vi "PathPlanner_Path_BezierFromPoses.vi"(11 "Poses":T2[](array[typedef]) {"ROTATION"."SIN" format="%13.4f"; "ROTATION"."COS" format="%13.4f"; "ROTATION"."VALUE" format="%13.4f"; "TRANSLATION"."Y" format="%14.3f"; "TRANSLATION"."X" format="%14.3f"}) -> (0 "Error":bool, 3 "Bezier":T1[](array[typedef]) {"Y" format="%14.3f"; "X" format="%14.3f"})   [LabVIEW 2019, in "PathPlanner24.lvlib"]
doc: "Create the bezier points necessary to create a path using a list of poses\n\nInputs: \n - poses - pose2d array - List of poses. Each pose represents one waypoint.\n\nOutputs:\n - Bezier - translation2d array - List of bezier points\n - Error - boolean - TRUE if an error occured. (Too few poses)"
uses:
  PathPlanner24.lvlib
  <vilib>/Rock Robotics/WPI/ThirdParty/JAS_Junk/TrajLib/TypeDef/POSE2D.ctl
  <vilib>/Rock Robotics/WPI/ThirdParty/JAS_Junk/TrajLib/TypeDef/TRANSLATION2D.ctl
  <vilib>/Rock Robotics/WPI/ThirdParty/JAS_Junk/TrajLib/TypeDef/ROTATION2D.ctl
  <vilib>/Rock Robotics/WPI/ThirdParty/JAS_Junk/TrajLib/Util_CalcDist.vi
  <vilib>/Rock Robotics/WPI/ThirdParty/JAS_Junk/TrajLib/Rotation2d_GetAngleCosSin.vi
  <vilib>/Rock Robotics/WPI/ThirdParty/JAS_Junk/TrajLib/Translation2d_Create.vi
  <vilib>/Rock Robotics/WPI/ThirdParty/JAS_Junk/TrajLib/Rotation2d_RotateBy.vi
  <vilib>/Rock Robotics/WPI/ThirdParty/JAS_Junk/TrajLib/Conv_Deg_Radians.vi
  <vilib>/Rock Robotics/WPI/ThirdParty/JAS_Junk/TrajLib/Rotation2d_CreateAngle.vi
  <vilib>/Rock Robotics/WPI/ThirdParty/JAS_Junk/TrajLib/Rotation2d_CreateXY.vi
  <vilib>/Rock Robotics/WPI/ThirdParty/JAS_Junk/TrajLib/Trajectory_Library.lvlib
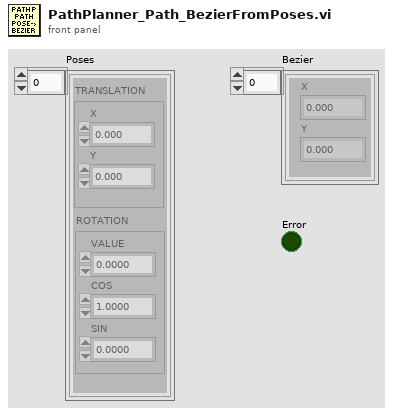
[diagram p1: front panel]
types:
  T1 = typedef "Trajectory_Library.lvlib/TRANSLATION2D.ctl" = cluster{"X":dbl, "Y":dbl}
  T2 = typedef "Trajectory_Library.lvlib/POSE2D.ctl" = cluster{"TRANSLATION":T1, "ROTATION":T3}
  T3 = typedef "Trajectory_Library.lvlib/ROTATION2D.ctl" = cluster{"VALUE":dbl, "COS":dbl, "SIN":dbl}
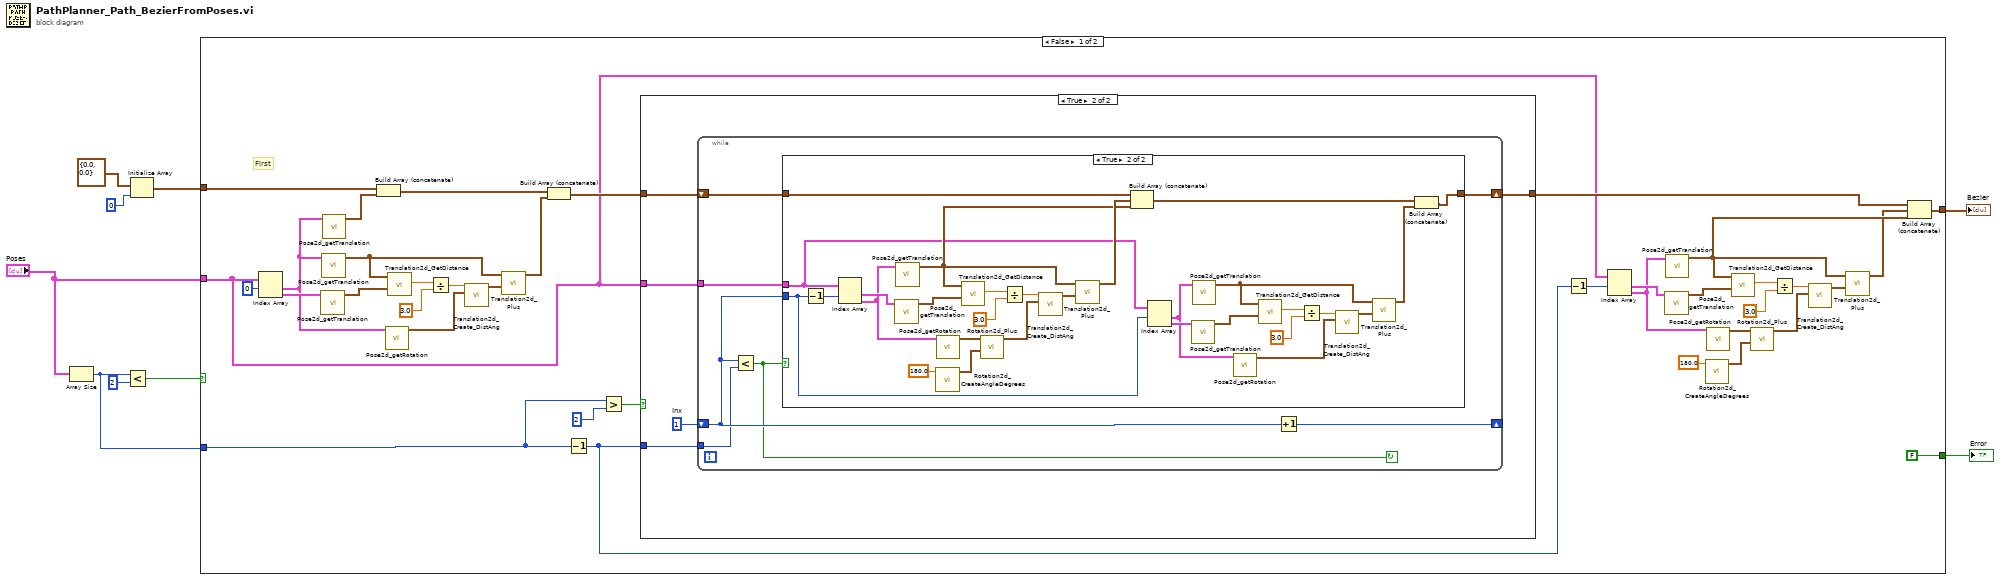
[diagram p0: block diagram]
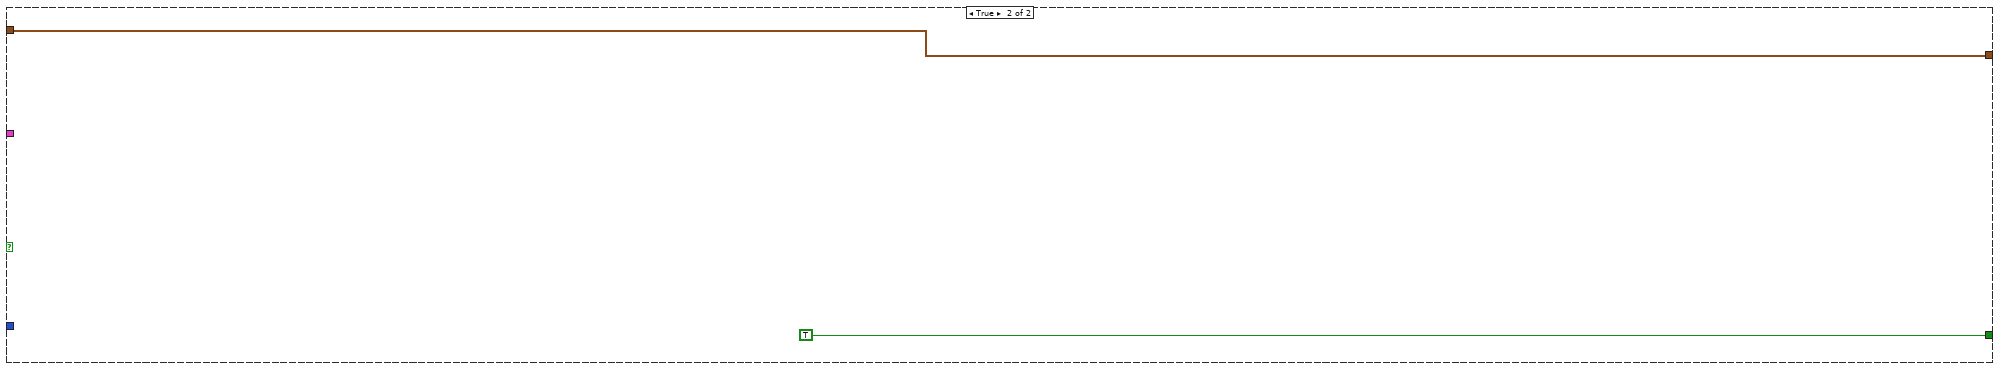
[diagram p4: hidden frame]
diagram:
  n1 = Array Size(array="Poses") -> (size(s)=w2:i32)
  n2 = Less?(x=w2, y=2) -> (x < y?=w6:bool)
  n3 = Initialize Array(T1 {"X"=0.0, "Y"=0.0} ("Bezier"), 0 ("dimension size")) -> (w5:T1[])
  n4 = case shown="False" w6 {
    tunnel: w5 -> [w46 w91]
    tunnel: [w19 w91] -> w1
    tunnel: [FALSE TRUE] -> w4
    tunnel: "Poses" -> [w18 _]
    tunnel: w2 -> [w11 _]
    frame False {
      # "First"
      n5 = Index Array(array=w18, index #1=0 ("index")) -> (element #1=w36:T2, element #2=w44:T2)  [unwired: 1 in]
      n6 = call <vilib>:"Pose2d_getTranslation.vi"("in POSE"=w44) -> ("outTRANSLATION"=w43:T1)  [unwired: 10 in]
      n7 = call <vilib>:"Pose2d_getTranslation.vi"("in POSE"=w36) -> ("outTRANSLATION"=w38:T1)  [unwired: 10 in]
      n8 = call <vilib>:"Pose2d_getTranslation.vi"("in POSE"=w36) -> ("outTRANSLATION"=w35:T1)  [unwired: 10 in]
      n9 = Build Array (concatenate)(w46, w35) -> (w34:T1[])
      n10 = call <vilib>:"Pose2d_getRotation.vi"("in POSE"=w36) -> ("out ROTATION"=w39:T3)  [unwired: 10 in]
      n11 = call <vilib>:"Translation2d_GetDistance.vi"("other Translation"=w43, "In Translation"=w38) -> ("Distance"=w42:dbl)  [unwired: 9 in]
      n12 = Divide(x=w42, y=3.0) -> (x/y=w40:dbl)
      n13 = call <vilib>:"Translation2d_Create_DistAng.vi"("Angle"=w39, "Dist"=w40) -> ("TRANSLATION"=w37:T1)  [unwired: 9 in]
      n14 = call <vilib>:"Translation2d_Plus.vi"("other Translation"=w37, "In Translation"=w38) -> ("Out Translation"=w33:T1)  [unwired: 9 in]
      n15 = Build Array (concatenate)(w34, w33) -> (w32:T1[])
      n16 = Decrement(x=w11) -> (x-1=w17:i32)
      n17 = Greater?(x=w11, y=2) -> (0:w12:bool)
      n18 = case shown="True" w12 {
        tunnel: w32 -> [w47 w52]
        tunnel: [w47 w50] -> w20
        tunnel: w18 -> [_ w49]
        tunnel: w17 -> [_ w48]
        frame False {
        }
        frame True {
          w51 = 1  # Inx
          n19 = while {
            shift-right: [w56] -> w50
            shift-left: w52 -> [w58]
            shift-right: [w59] -> _
            shift-left: w51 -> [w55]
            tunnel: w49 -> [w57]
            tunnel: w48 -> [w54]
            stop <- w53 continue-if-true
            n20 = Less?(x=w55, y=w54) -> (x < y?=w53:bool)
            n21 = case shown="True" w53 {
              tunnel: w58 -> [w60 w77]
              tunnel: w57 -> [_ w68]
              tunnel: w55 -> [_ w61]
              tunnel: [w60 w62] -> w56
              frame False {
              }
              frame True {
                n22 = Decrement(x=w61) -> (x-1=w89:i32)
                n23 = Index Array(array=w68, index #1=w89) -> (element #1=w83:T2, element #2=w80:T2)  [unwired: 1 in]
                n24 = call <vilib>:"Pose2d_getTranslation.vi"("in POSE"=w83) -> ("outTRANSLATION"=w88:T1)  [unwired: 10 in]
                n25 = call <vilib>:"Pose2d_getTranslation.vi"("in POSE"=w80) -> ("outTRANSLATION"=w75:T1)  [unwired: 10 in]
                n26 = call <vilib>:"Rotation2d_CreateAngleDegrees.vi"("Angle_Degrees"=180.0) -> ("ROTATION"=w78:T3)  [unwired: 10 in]
                n27 = call <vilib>:"Pose2d_getRotation.vi"("in POSE"=w80) -> ("out ROTATION"=w82:T3)  [unwired: 10 in]
                n28 = call <vilib>:"Translation2d_GetDistance.vi"("other Translation"=w88, "In Translation"=w75) -> ("Distance"=w87:dbl)  [unwired: 9 in]
                n29 = call <vilib>:"Rotation2d_Plus.vi"("other ROTATION"=w78, "in ROTATION"=w82) -> ("out ROTATION"=w81:T3)  [unwired: 9 in]
                n30 = Divide(x=w87, y=3.0) -> (x/y=w85:dbl)
                n31 = call <vilib>:"Translation2d_Create_DistAng.vi"("Angle"=w81, "Dist"=w85) -> ("TRANSLATION"=w84:T1)  [unwired: 9 in]
                n32 = call <vilib>:"Translation2d_Plus.vi"("other Translation"=w84, "In Translation"=w75) -> ("Out Translation"=w76:T1)  [unwired: 9 in]
                n33 = Build Array (concatenate)(w77, w76, w75) -> (w64:T1[])
                n34 = Index Array(array=w68, index #1=w61) -> (element #1=w65:T2, element #2=w67:T2)  [unwired: 1 in]
                n35 = call <vilib>:"Pose2d_getTranslation.vi"("in POSE"=w67) -> ("outTRANSLATION"=w74:T1)  [unwired: 10 in]
                n36 = call <vilib>:"Pose2d_getTranslation.vi"("in POSE"=w65) -> ("outTRANSLATION"=w69:T1)  [unwired: 10 in]
                n37 = call <vilib>:"Pose2d_getRotation.vi"("in POSE"=w65) -> ("out ROTATION"=w66:T3)  [unwired: 10 in]
                n38 = call <vilib>:"Translation2d_GetDistance.vi"("other Translation"=w74, "In Translation"=w69) -> ("Distance"=w73:dbl)  [unwired: 9 in]
                n39 = Divide(x=w73, y=3.0) -> (x/y=w71:dbl)
                n40 = call <vilib>:"Translation2d_Create_DistAng.vi"("Angle"=w66, "Dist"=w71) -> ("TRANSLATION"=w70:T1)  [unwired: 9 in]
                n41 = call <vilib>:"Translation2d_Plus.vi"("other Translation"=w70, "In Translation"=w69) -> ("Out Translation"=w63:T1)  [unwired: 9 in]
                n42 = Build Array (concatenate)(w64, w63) -> (w62:T1[])
              }
            }
            n43 = Increment(x=w55) -> (x+1=w59:i32)
          }
        }
      }
      n44 = Decrement(x=w17) -> (x-1=w16:i32)
      n45 = Index Array(array=w18, index #1=w16) -> (element #1=w26:T2, element #2=w23:T2)  [unwired: 1 in]
      n46 = call <vilib>:"Pose2d_getTranslation.vi"("in POSE"=w26) -> ("outTRANSLATION"=w31:T1)  [unwired: 10 in]
      n47 = call <vilib>:"Pose2d_getTranslation.vi"("in POSE"=w23) -> ("outTRANSLATION"=w15:T1)  [unwired: 10 in]
      n48 = call <vilib>:"Rotation2d_CreateAngleDegrees.vi"("Angle_Degrees"=180.0) -> ("ROTATION"=w21:T3)  [unwired: 10 in]
      n49 = call <vilib>:"Pose2d_getRotation.vi"("in POSE"=w23) -> ("out ROTATION"=w25:T3)  [unwired: 10 in]
      n50 = call <vilib>:"Translation2d_GetDistance.vi"("other Translation"=w31, "In Translation"=w15) -> ("Distance"=w30:dbl)  [unwired: 9 in]
      n51 = call <vilib>:"Rotation2d_Plus.vi"("other ROTATION"=w21, "in ROTATION"=w25) -> ("out ROTATION"=w24:T3)  [unwired: 9 in]
      n52 = Divide(x=w30, y=3.0) -> (x/y=w28:dbl)
      n53 = call <vilib>:"Translation2d_Create_DistAng.vi"("Angle"=w24, "Dist"=w28) -> ("TRANSLATION"=w27:T1)  [unwired: 9 in]
      n54 = call <vilib>:"Translation2d_Plus.vi"("other Translation"=w27, "In Translation"=w15) -> ("Out Translation"=w14:T1)  [unwired: 9 in]
      n55 = Build Array (concatenate)(w20, w14, w15) -> (w19:T1[])
    }
    frame True {
    }
  }
  "Bezier" <- w1
  "Error" <- w4
